vi "Convert OpenCV to IMAQ.vi"() -> ()   [LabVIEW 2017]
uses:
  IMAQCV/IMAQCV.lvlib
panel:
  out "error out":errorcluster
  out "Image":T1(plugin-control)
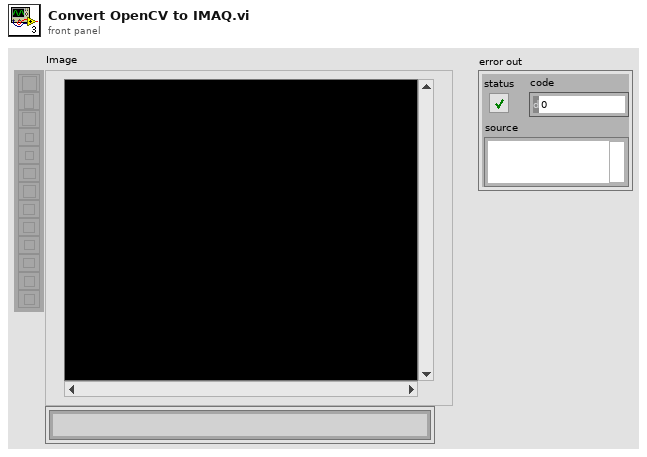
[diagram p1: front panel]
types:
  T1 = typedef "IMAQ Image.ctl" = refnum<image>
  T2 = enum16{"320 (H)   x  240 (V)", "352(H)    x  288 (V)", "640 (H)   x  480 (V) ", "800 (H)   x  600 (V)", "1024 (H) x  768 (V)", "1280 (H) x  720 (V)", "1280 (H) x  960 (V)", "1280 (H) x 1024 (V)", "1920 (H) x 1080 (V)"}
  T3 = typedef "Image Type" = u32
  T4 = typedef "IMAQCV.lvlib/IMAQCV Image.ctl" = refnum<vi>
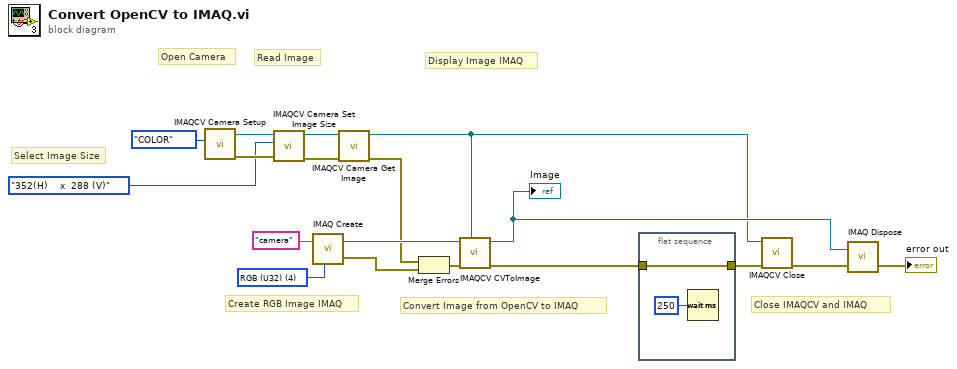
[diagram p0: block diagram]
diagram:
  w13 = T3 4 items=["Grayscale (U8)", "Grayscale (I16)", "Grayscale (SGL)", "Complex (CSG)", "RGB (U32)", "HSL (U32)", "RGB (U64)", "Grayscale (U16)"] ("Image Type")
  # "Close IMAQCV and IMAQ"
  # "Convert Image from OpenCV to IMAQ"
  # "Create RGB Image IMAQ"
  # "Display Image IMAQ"
  # "Select Image Size"
  # "Read Image"
  # "Open Camera"
  n1 = call "IMAQCV Camera Setup.vi"("type"=enum16{"GRAY", "COLOR"}."COLOR") -> ("error out"=w16:errorcluster, "image out"=w15:T4)  [unwired: 9 in]
  n2 = call "IMAQCV Camera Set Image Size.vi"("error in (no error)"=w16, "Image Size"=T2."352(H)    x  288 (V)", "image in"=w15) -> ("error out"=w18:errorcluster, "image out"=w17:T4)  [unwired: 7 in]
  n3 = call "IMAQ Create"("Image Name"="camera", "Image Type"=w13) -> ("New Image"=w12:T1, "error out"=w4:errorcluster)  [unwired: 2 in, 1 out]
  n4 = call "IMAQCV Camera Get Image.vi"("error in (no error)"=w18, "image in"=w17) -> ("error out"=w5:errorcluster, "image out"=w10:T4)  [unwired: 8 in]
  n5 = Merge Errors(w5, w4) -> (w3:errorcluster)
  n6 = call "IMAQCV CVToImage.vi"("cvimage in"=w10, "error in (no error)"=w3, "Variant In"=w12) -> ("error out"=w2:errorcluster, "Variant Out"=w11:refnum<image>)  [unwired: 7 in]
  "Image" <- w11
  n7 = flat-sequence {
    tunnel: w2 -> [w20]
    tunnel: [w20] -> w1
    frame #0 {
      n8 = Wait (ms)(milliseconds to wait=u32 250) -> ()  [unwired: 1 out]
    }
  }
  n9 = call "IMAQCV Close.vi"("error in (no error)"=w1, "Image"=w10) -> ("error out"=w8:errorcluster)  [unwired: 9 in]
  n10 = call "IMAQ Dispose"("Image"=w11, "error in (no error)"=w8) -> ("error out"=→"error out":errorcluster)  [unwired: 4 in]
